vi "Actor Core.vi"(8 "error in":errorcluster, 11 "GUI View in":refnum<class "GUI View.lvclass">) -> (0 "error out":errorcluster, 3 "Actor out":refnum<class "Actor.lvclass">)   [LabVIEW 2023, in "GUI Views.lvlib" / "GUI View.lvclass"]
doc: "(<B>Filename</B>: Actor Framework.lvlib:Actor.lvclass:Actor Core.vi)\n\nReceives messages to the actor, reacts to them, and initiates any error handling that may shut the actor down.\n\nDescendant classes may override this VI to append parallel tasks for the actor to complete while it handles messages. Overrides use the Call Parent Method node."
uses:
  GUI View.lvclass
  View/View.lvclass
  <vilib>/ActorFramework/Actor/Actor.lvclass
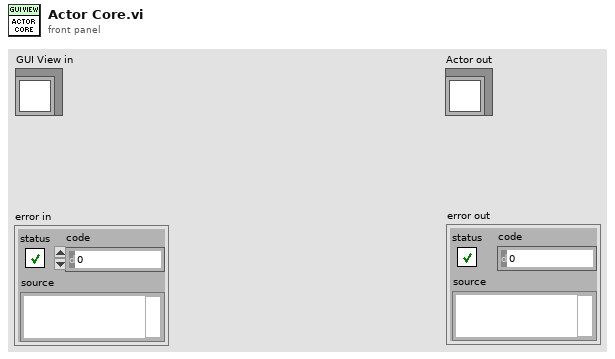
[diagram p1: front panel]
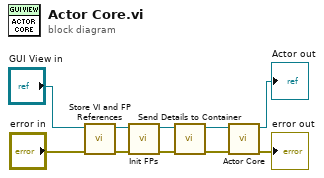
[diagram p0: block diagram]
diagram:
  n1 = call "Store VI and FP References.vi"("error in (no error)"="error in", "GUI View in"="GUI View in") -> ("error out"=w3:errorcluster, "GUI View out"=w4:refnum<class "GUI View.lvclass">)  [unwired: 8 in]
  n2 = call-dynamic "Init FPs.vi"("error in (no error)"=w3, "GUI View in"=w4) -> ("error out"=w2:errorcluster, "GUI View out"=w1:refnum<class "GUI View.lvclass">)  [unwired: 8 in]
  n3 = call "Send Details to Container.vi"("error in (no error)"=w2, "GUI View in"=w1) -> ("error out"=w6:errorcluster, "GUI View out"=w5:refnum<class "GUI View.lvclass">)  [unwired: 8 in]
  n4 = call-parent "Actor Core.vi"("error in"=w6, "Actor in"=w5) -> ("error out"=→"error out":errorcluster, "Actor out"=→"Actor out":refnum<class "Actor.lvclass">)  [unwired: 8 in]
